vi "Problem 18.vi"() -> ()   [LabVIEW 2013, in "Problem 18.lvlib"]
uses:
  Problem 18.lvlib
panel:
  out "max value":u32
  in  "# Pyramid":string="75\n95 64\n17 47 82\n18 35 87 10\n20 04 82 47 65\n19 01 23 75 03 34\n88 02 77 73 07 63 67\n99 65 04 28 06 16 70 92\n41 41 26 56 83 40 80 70 33\n41 48 72 33 47 32 37 16 94 29\n53 71 44 65 25 43 91 52 97 51 14\n70 11 33 28 77 73 17 78 39 68 17 57\n91 71 52 38 17 14 91 43 58 50 27 29 48\n63 66 04 68 89 53 67 30 73 16 69 87 40 31\n04 62 98 27 23 09 70 98 73 93 38 53 60 04 23"
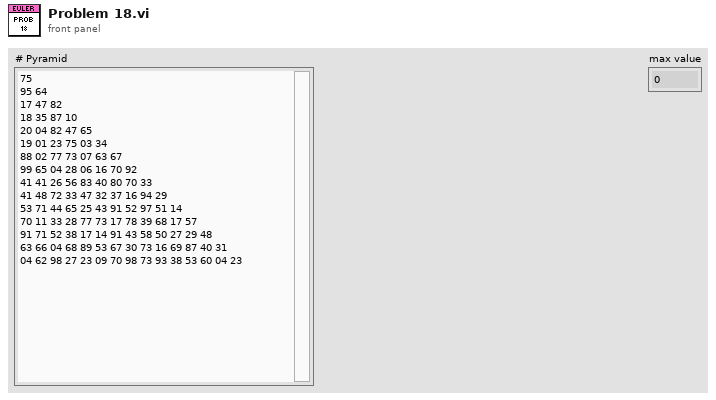
[diagram p1: front panel]
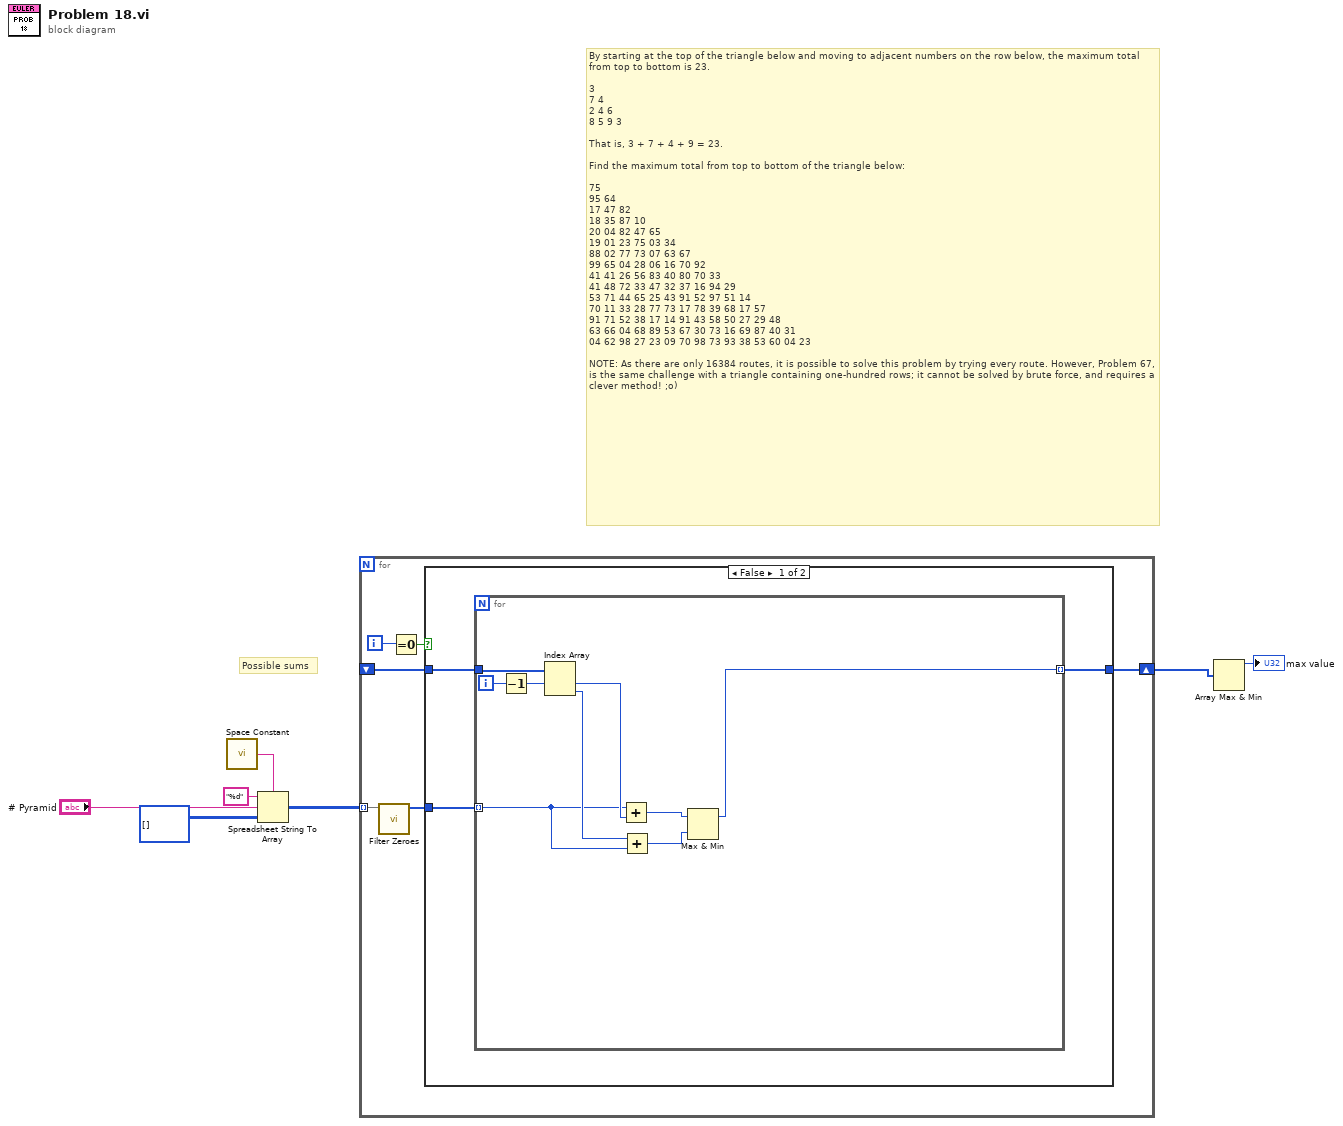
[diagram p0: block diagram]
diagram:
  # "Possible sums"
  # "By starting at the top of the triangle below and moving to adjacent numbers on the row below, the maximum total from top to bottom is 23.\n\n3\n7 4\n2 4 6\n8 5 9 3\n\nThat is, 3 + 7 + 4 + 9 = 23.\n\nFind the maximum total from top to bottom of the triangle below:\n\n75\n95 64\n17 47 82\n18 35 87 10\n20 04 82 47 65\n19 01 23 75 03 34\n88 02 77 73 07 63 67\n99 65 04 28 06 16 70 92\n41 41 26 56 83 40 80 70 33\n41 48 72 33 47 32 37 16 94 29\n53 71 44 65 25 43 91 52 97 51 14\n70 11 33 28 77 73 17 78 39 68 17 57\n91 71 52 38 17 14 91 43 58 50 27 29 48\n63 66 04 68 89 53 67 30 73 16 69 87 40 31\n04 62 98 27 23 09 70 98 73 93 38 53 60 04 23\n\nNOTE: As there are only 16384 routes, it is possible to solve this problem by trying every route. However, Problem 67, is the same challenge with a triangle containing one-hundred rows; it cannot be solved by brute force, and requires a clever method! ;o)"
  n1 = call <vilib>:"Space Constant.vi"() -> ("String"=w4:string)
  n2 = Spreadsheet String To Array(delimiter (Tab)=w4, format string="%d", spreadsheet string="# Pyramid", array type (2D Dbl)=u32[][] []) -> (array=w3:u32[][])
  n3 = for {
    tunnel: w3 -> [w11] mode=indexing
    shift-right: [w10] -> w2
    shift-left: _ -> [w9]
    i -> [w13]
    n4 = call "Filter Zeroes.vi"("Array in"=w11) -> ("Array out"=w8:u32[])  [unwired: 10 in]
    n5 = Equal To 0?(x=w13) -> (x = 0?=w12:bool)
    n6 = case shown="False" w12 {
      tunnel: w8 -> [w16 w26]
      tunnel: [w14 w26] -> w10
      tunnel: w9 -> [w15 _]
      frame False {
        n7 = for {
          tunnel: w16 -> [w21] mode=indexing
          tunnel: w15 -> [w25]
          tunnel: [w18] -> w14 mode=indexing
          i -> [w24]
          n8 = Decrement(x=w24) -> (x-1=w17:i32)
          n9 = Index Array(array=w25, index #1=w17) -> (element #1=w23:u32, element #2=w22:u32)  [unwired: 1 in]
          n10 = Add(x=w21, y=w23) -> (x+y=w20:u32)
          n11 = Add(x=w22, y=w21) -> (x+y=w19:u32)
          n12 = Max & Min(x=w20, y=w19) -> (max(x,y)=w18:u32)  [unwired: 1 out]
        }
      }
      frame True {
      }
    }
  }
  n13 = Array Max & Min(array=w2) -> (max value=→"max value":u32)  [unwired: 3 out]
